vi "GV_YscaleDelete.vi"(8 "error in (no error)":errorcluster, 9 "Plot":i32, 11 "Gviewer in":refnum<class "Gviewer.lvclass">) -> (0 "error out":errorcluster, 3 "Gviewer out":refnum<class "Gviewer.lvclass">)   [LabVIEW 2020, in "Sgraph_lib_V1.lvlib" / "Gviewer.lvclass"]
doc: "Remoe one Y-scale from graph"
uses:
  Gviewer.lvclass
  Gviewer.lvclass/Gviewer.ctl
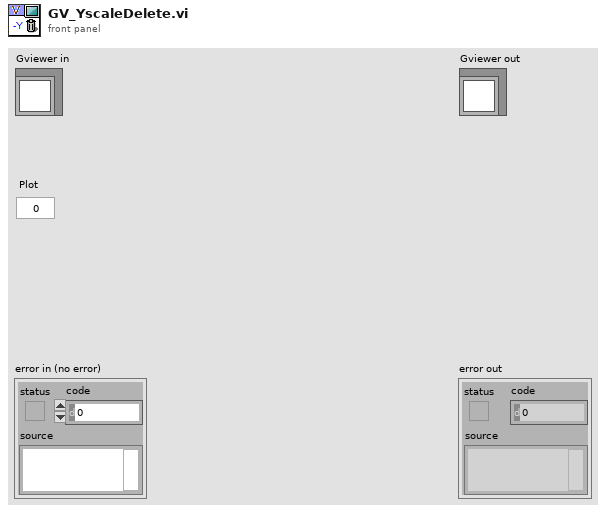
[diagram p1: front panel]
types:
  T1 = typedef "Sgraph_lib_V1.lvlib/Gviewer.lvclass/YgraphDef.ctl" = cluster{"Plot":i32, "X(%)":dbl}
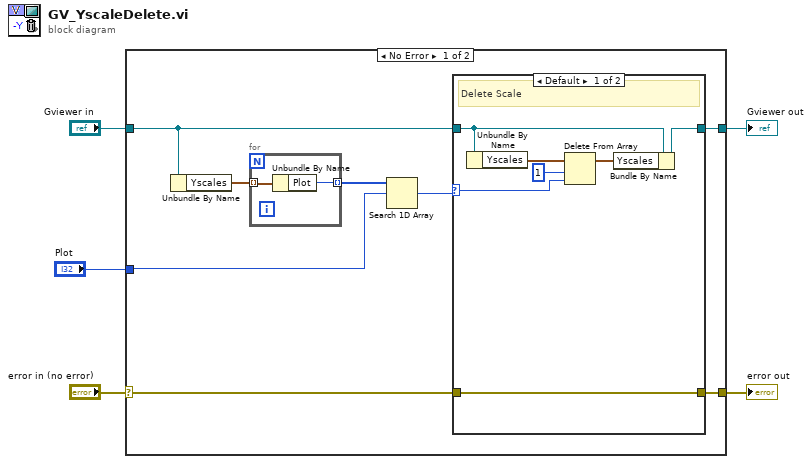
[diagram p0: block diagram]
diagram:
  n1 = case shown="No Error" "error in (no error)" {
    selector: "error in (no error)" -> [w11 w26]
    tunnel: [w9 w26] -> w4
    tunnel: [w10 w25] -> w2
    tunnel: "Gviewer in" -> [w12 w25]
    tunnel: "Plot" -> [w7 _]
    frame No Error {
      n2 = Unbundle By Name(w12) -> ("Yscales"=w13:T1[])
      n3 = for {
        tunnel: w13 -> [w24] mode=indexing
        tunnel: [w23] -> w8 mode=indexing
        n4 = Unbundle By Name(w24) -> ("Plot"=w23:i32)
      }
      n5 = Search 1D Array(1D array=w8, element=w7) -> (index of element=w6:i32)  [unwired: 1 in]
      n6 = case shown="Default" w6 {
        selector: w6 -> [w18 _]
        tunnel: w12 -> [w17 w22]
        tunnel: w11 -> [w14 w21]
        tunnel: [w15 w22] -> w10
        tunnel: [w14 w21] -> w9
        frame Default {
          # "Delete Scale"
          n7 = Unbundle By Name(w17) -> ("Yscales"=w20:T1[])
          n8 = Delete From Array(array=w20, length=1, index=w18) -> (array with subset deleted=w16:T1[])  [unwired: 1 out]
          n9 = Bundle By Name(cluster=w17, "Yscales"=w16) -> (w15:refnum<class "Gviewer.lvclass">)
        }
        frame -1 {
          # "Not found"
        }
      }
    }
    frame Error {
    }
  }
  "error out" <- w4
  "Gviewer out" <- w2
